vi "SDCP SMF Transmitter and Receiver - Generate Plot Files from Trace Files.vi"(6 "error in (no error)":errorcluster, 7 "Trace File Path":path=path "E:/Projects/System Diagnostics and Control Protocol/SDCP_LabVIEW/temp/Trace Files/TRACE_14_05_2024__00_15_13/0.csv", 10 "Parameter file path":path=path "E:/Projects/System Diagnostics and Control Protocol/SDCP_LabVIEW/Parameter Files/Motion_Processing.param") -> (0 "error out":errorcluster)   [LabVIEW 2020]
uses:
  <vilib>/Utility/file.llb/Write Delimited Spreadsheet (string).vi
panel:
  out "File counter":i32
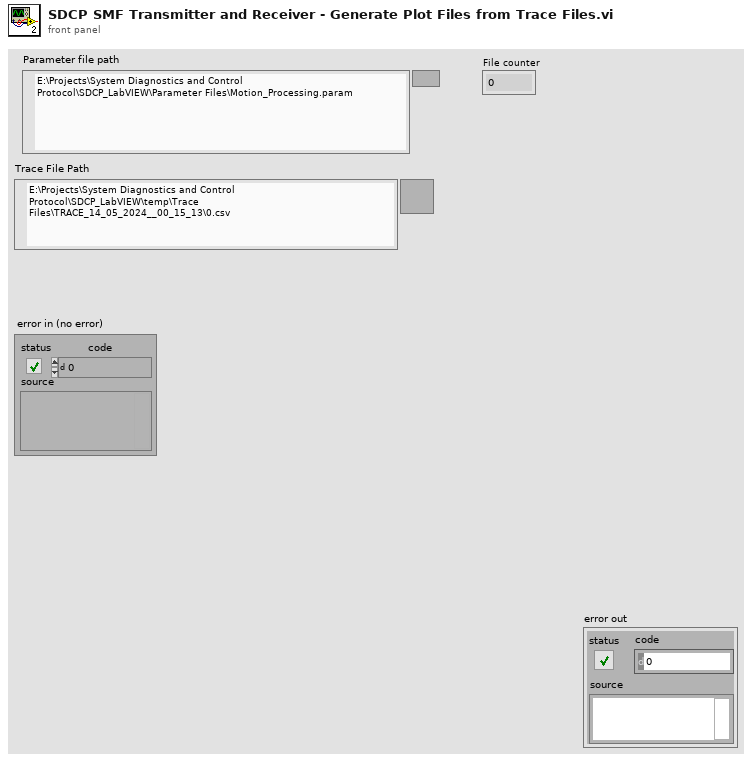
[diagram p1: front panel]
types:
  T1 = enum16{"open", "replace", "create", "open or create", "replace or create", "replace or create with confirmation"}
  T2 = cluster{"Plot data":cluster{"X":dbl, "Y":dbl}[], "Plot name":string}[]
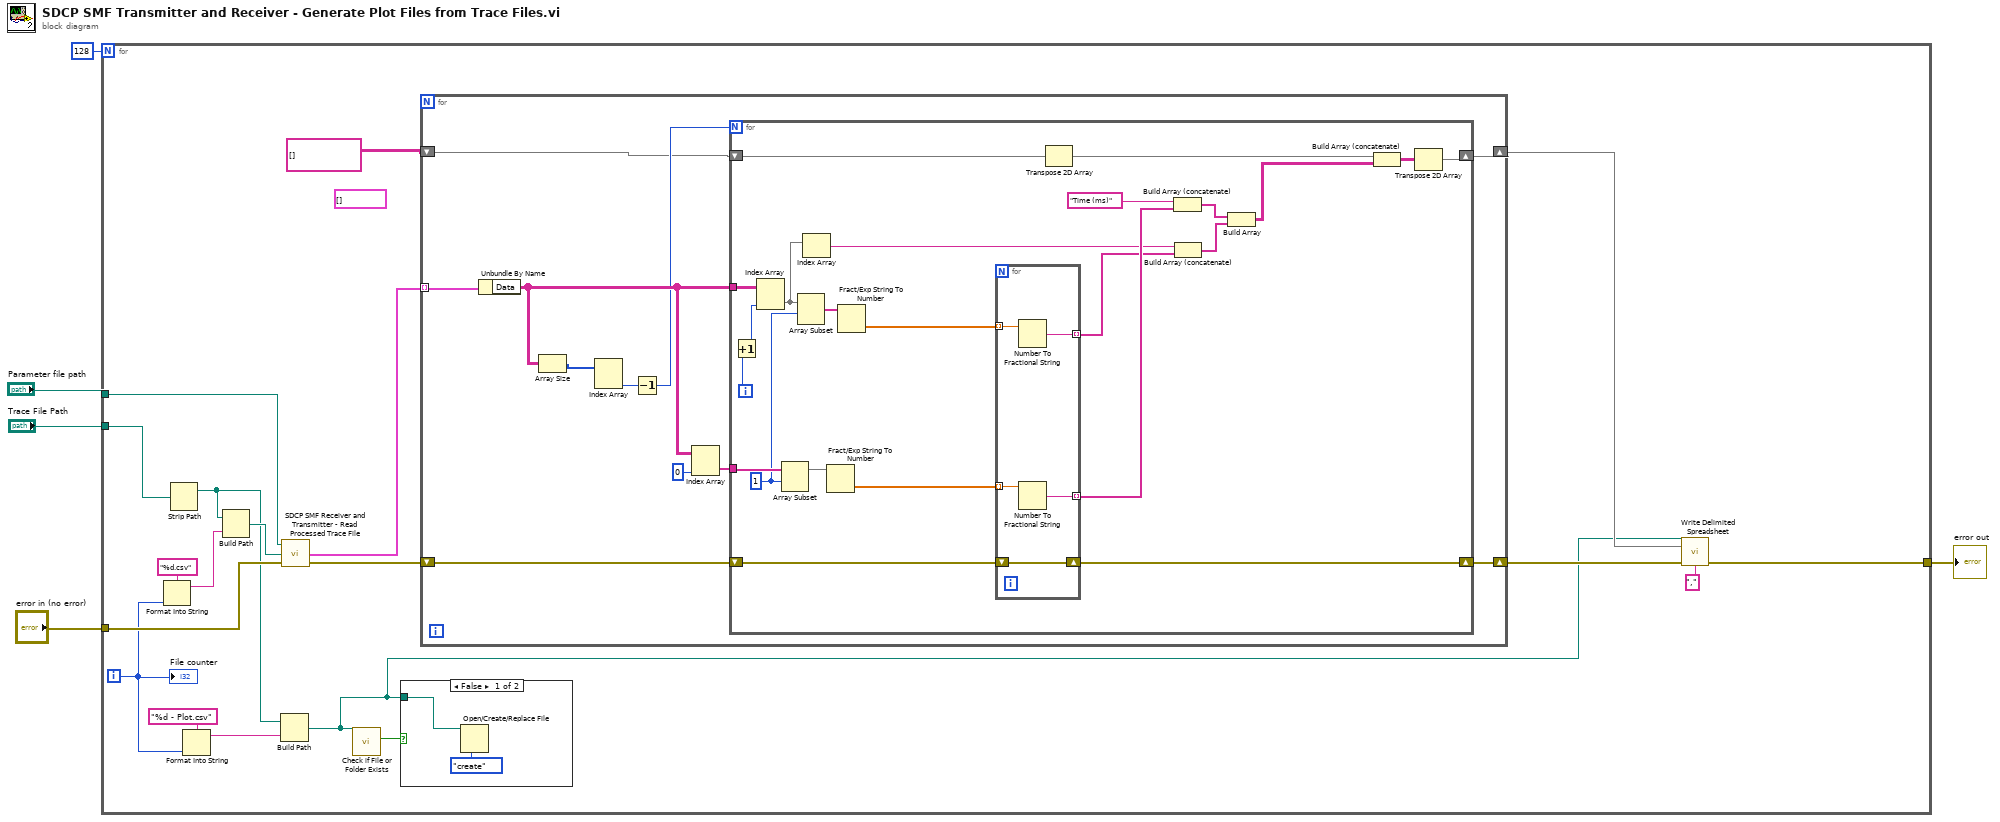
[diagram p0: block diagram]
diagram:
  n1 = for {
    N: 128 -> [_]
    tunnel: "Parameter file path" -> [w24]
    tunnel: "Trace File Path" -> [w20]
    tunnel: "error in (no error)" -> [w23]
    tunnel: [w11] -> w2
    i -> [w15]
    (unwired) T2 []
    n2 = Format Into String(format string="%d.csv", w15) -> (resulting string=w18:string)  [unwired: 2 in, 1 out]
    n3 = Strip Path(path=w20) -> (stripped path=w6:path)  [unwired: 1 out]
    n4 = Format Into String(format string="%d - Plot.csv", w15) -> (resulting string=w14:string)  [unwired: 2 in, 1 out]
    n5 = Build Path(base path=w6, name or relative path=w18) -> (appended path=w9:path)
    n6 = Build Path(base path=w6, name or relative path=w14) -> (appended path=w7:path)
    n7 = call "SDCP SMF Receiver and Transmitter - Read Processed Trace File.vi"("error in (no error)"=w23, "Trace File Path"=w9, "Parameter file path"=w24) -> ("error out"=w22:errorcluster, "Framewise output"=w21:cluster{"Data":string[][]}[])  [unwired: 1 out]
    n8 = call <vilib>:"Check if File or Folder Exists.vi"("path"=w7) -> ("file or folder exists?"=w13:bool)  [unwired: 8 in, 2 out]
    n9 = case shown="False" w13 {
      tunnel: w7 -> [w26 _]
      frame False {
        n10 = Open/Create/Replace File(file path (use dialog)=w26, operation (0:open)=T1."create") -> ()  [unwired: 4 in, 3 out]
      }
      frame True {
      }
    }
    n11 = for {
      shift-right: [w30] -> w12
      shift-left: w22 -> [w34]
      tunnel: w21 -> [w37] mode=indexing
      shift-right: [w27] -> w8
      shift-left: string[][] [] -> [w28]
      n12 = Unbundle By Name(w37) -> ("Data"=w33:string[][])
      n13 = Array Size(array=w33) -> (size(s)=w36:i32[])
      n14 = Index Array(array=w36) -> (element #2=w35:i32)  [unwired: 2 in, 1 out]
      n15 = Decrement(x=w35) -> (x-1=w32:i32)
      n16 = Index Array(array=w33, index (col)=0 ("disabled index (col)")) -> (element=w31:string[])  [unwired: 1 in]
      n17 = for {
        N: w32 -> [_]
        shift-right: [w50] -> w30
        shift-left: w34 -> [w51]
        tunnel: w33 -> [w60]
        tunnel: w31 -> [w56]
        shift-right: [w38] -> w27
        shift-left: w28 -> [w41]
        i -> [w59]
        w53 = 1 ("index")
        n18 = Increment(x=w59) -> (x+1=w49:i32)
        n19 = Index Array(array=w60, index (col)=w49) -> (element=w52:string[])  [unwired: 1 in]
        n20 = Array Subset(array=w56, index=w53) -> (w55:string[])  [unwired: 1 in]
        n21 = Array Subset(array=w52, index=w53) -> (w54:string[])  [unwired: 1 in]
        n22 = Index Array(array=w52) -> (element=w46:string)  [unwired: 1 in]
        n23 = Fract/Exp String To Number(string=w55) -> (number=w57:dbl[])  [unwired: 3 in, 1 out]
        n24 = Fract/Exp String To Number(string=w54) -> (number=w58:dbl[])  [unwired: 3 in, 1 out]
        n25 = for {
          tunnel: w58 -> [w64] mode=indexing
          tunnel: w57 -> [w63] mode=indexing
          shift-right: [w65] -> w50
          shift-left: w51 -> [w65]
          tunnel: [w62] -> w45 mode=indexing
          tunnel: [w61] -> w47 mode=indexing
          n26 = Number To Fractional String(number=w64) -> (F-format string=w62:string)  [unwired: 3 in]
          n27 = Number To Fractional String(number=w63) -> (F-format string=w61:string)  [unwired: 3 in]
        }
        n28 = Transpose 2D Array(2D array=w41) -> (transposed array=w39:string[][])
        n29 = Build Array (concatenate)("Time (ms)" ("element"), w47) -> (w44:string[])
        n30 = Build Array (concatenate)(w46, w45) -> (w43:string[])
        n31 = Build Array(w44, w43) -> (w42:string[][])
        n32 = Build Array (concatenate)(w39, w42) -> (w40:string[][])
        n33 = Transpose 2D Array(2D array=w40) -> (transposed array=w38:string[][])
      }
    }
    n34 = call-poly <vilib>:"Write Delimited Spreadsheet.vi"("file path (dialog if empty)"=w7, "2D data"=w8, "error in (no error)"=w12, "delimiter (\\t)"="," ("delimiter (\\t)")) -> ("error out"=w11:errorcluster)  [unwired: 10 in, 1 out]
    "File counter" <- w15
  }
  "error out" <- w2
